vi "Get Channel Auxiliary Data Type.vi"(8 "error in":errorcluster, 11 "Plugin_Controller in":refnum<class "Plugin_Controller.lvclass">) -> (0 "error out":errorcluster, 2 "Channel Auxiliary Data Type":variant, 3 "Plugin_Controller out":refnum<class "Plugin_Controller.lvclass">)   [LabVIEW 2020, in "Plugin.lvlib" / "Plugin_Controller.lvclass"]
doc: "Reads the channel's Auxiliary data type"
uses:
  Plugin_Controller.lvclass
  UI_Class/Auxiliary Data.ctl
  Channels/Plugin_Channels.lvclass
  UI_Class/Plugin_UI.lvclass
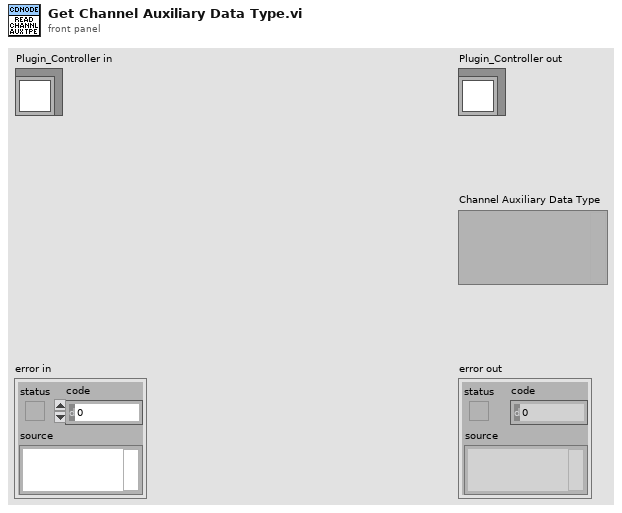
[diagram p1: front panel]
types:
  T1 = typedef "Plugin.lvlib/Plugin_UI.lvclass/Auxiliary Data.ctl" = cluster{"Plugin_Data":refnum<class "Plugin_Channels.lvclass">}
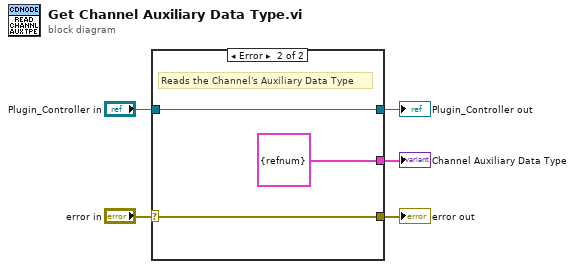
[diagram p0: block diagram]
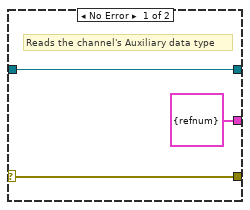
[diagram p2: hidden frame]
diagram:
  n1 = case shown="Error" "error in" {
    selector: "error in" -> [w7 w10]
    tunnel: "Plugin_Controller in" -> [w8 w11]
    tunnel: [T1 {"Plugin_Data"=refnum} ("Auxiliary Data") T1 {"Plugin_Data"=refnum} ("Auxiliary Data")] -> w3
    tunnel: [w8 w11] -> w2
    tunnel: [w7 w10] -> w1
    frame No Error {
      # "Reads the channel's Auxiliary data type"
    }
    frame Error {
      # "Reads the Channel's Auxiliary Data Type"
    }
  }
  "error out" <- w1
  "Plugin_Controller out" <- w2
  "Channel Auxiliary Data Type" <- w3
